vi "Extract Element Names.vi"(9 "Parent Name":string, 10 "Name (empty: Type label)":string, 11 "Type":variant) -> (1 "Default Values":variant[](array[variant]), 2 "Names":string[](array[string]), 3 "Type dup":variant)   [LabVIEW 2013]
uses:
  <vilib>/Utility/VariantDataType/VariantType.lvlib
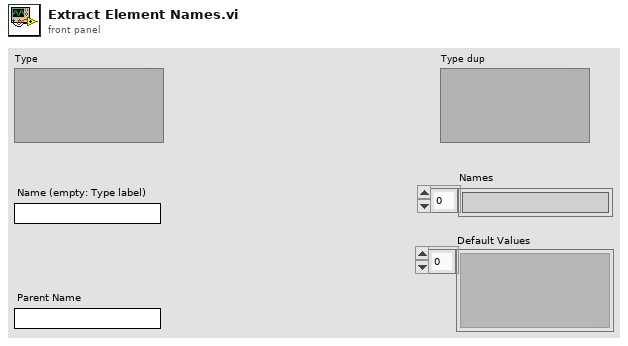
[diagram p1: front panel]
types:
  T1 = typedef "VariantType.lvlib/Type.ctl" = enum8{"Invalid Type", "Void", "I8", "I16", "I32", "I64", "U8", "U16", "U32", "U64", "Single Float", "Double Float", "Extended Float", "Single Complex", "Double Complex", "Extended Complex", "Enum U8", "Enum U16", "Enum U32", "Enum U64", "Single Float With Unit", "Double Float With Unit", "Extended Float With Unit", "Single Complex with Unit", "Double Complex with Unit", "Extended Complex with Unit", "Boolean", "String", "Path", "Picture", "Tag", "Array", "Cluster", "Variant", "LV Variant", "Waveform", "Timestamp", "Digital Waveform", "Digital Data", "ExpressData", "Refnum", "External Data", "VI", "Poly VI", "LabVIEW Class Instance", "Fixed Point"}
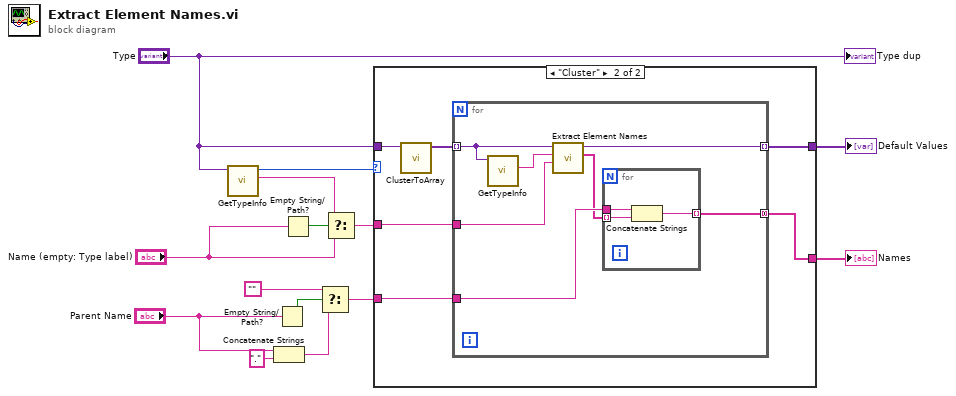
[diagram p0: block diagram]
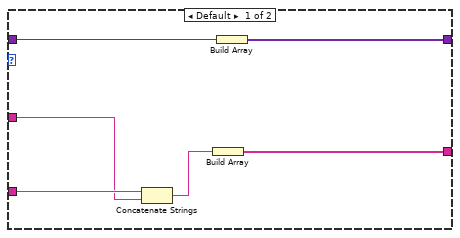
[diagram p2: hidden frame]
diagram:
  n1 = call <vilib>:"GetTypeInfo.vi"("Variant"="Type") -> ("Name"=w9:string, "Type Enum"=w14:T1)  [unwired: 6 in, 3 out]
  n2 = Concatenate Strings("Parent Name", "." ("string")) -> (w5:string)
  n3 = Empty String/Path?(string/path="Parent Name") -> (empty?=w8:bool)
  n4 = Empty String/Path?(string/path="Name (empty: Type label)") -> (empty?=w12:bool)
  n5 = Select(t="", s=w8, f=w5) -> (s? t:f=w3:string)
  n6 = Select(t=w9, s=w12, f="Name (empty: Type label)") -> (s? t:f=w10:string)
  n7 = case shown="\"Cluster\"" w14 {
    tunnel: "Type" -> [w16 w23]
    tunnel: w10 -> [w19 w25]
    tunnel: w3 -> [w20 w26]
    tunnel: [w17 w24] -> w2
    tunnel: [w15 w21] -> w1
    frame Default {
      n8 = Concatenate Strings(w20, w19) -> (w18:string)
      n9 = Build Array(w18) -> (w17:string[])
      n10 = Build Array(w16) -> (w15:variant[])
    }
    frame "Cluster" {
      n11 = call "ClusterToArray.vi"("Cluster"=w23) -> ("Array"=w22:variant[])  [unwired: 10 in]
      n12 = for {
        tunnel: w22 -> [w32] mode=indexing
        tunnel: w26 -> [w30]
        tunnel: w25 -> [w31]
        tunnel: [w28] -> w24 mode=concatenating
        tunnel: [w27] -> w21 mode=indexing
        n13 = call <vilib>:"GetTypeInfo.vi"("Variant"=w32) -> ("Name"=w33:string)  [unwired: 6 in, 4 out]
        n14 = call "Extract Element Names.vi"("Parent Name"=w31, "Name (empty: Type label)"=w33, "Type"=w32) -> ("Names"=w29:string[], "Type dup"=w27:variant)  [unwired: 6 in, 1 out]
        n15 = for {
          tunnel: w30 -> [w36]
          tunnel: w29 -> [w35] mode=indexing
          tunnel: [w34] -> w28 mode=indexing
          n16 = Concatenate Strings(w36, w35) -> (w34:string)
        }
      }
    }
  }
  "Names" <- w2
  "Default Values" <- w1
  "Type dup" <- "Type"
